vi "Log message.vi"(8 "error in (no error)":errorcluster, 9 "log level":u16(ring) items=[" STATUS ", " DEBBUG ", "  INFO  ", "WARNING ", " ERROR  ", "CRITICAL"], 10 "String":string, 11 "Channel in":refnum<class "Channel.lvclass">) -> (0 "error out":errorcluster, 3 "Channel out":refnum<class "Channel.lvclass">)   [LabVIEW 2018, in "Channel.lvclass"]
uses:
  Channel.lvclass
  Channel.lvclass/Channel.ctl
  Log File/Log File.lvclass
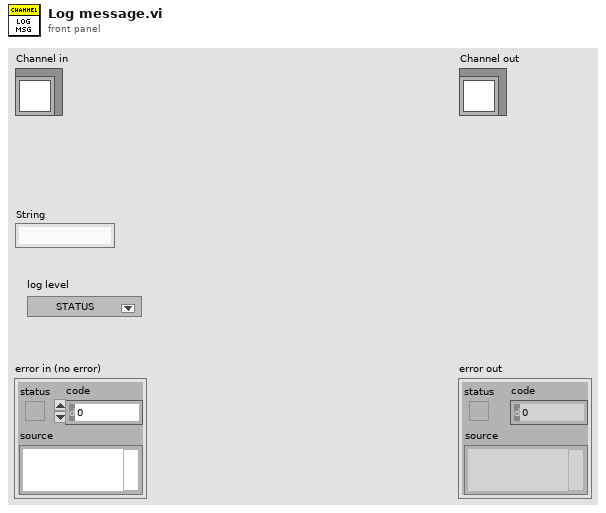
[diagram p1: front panel]
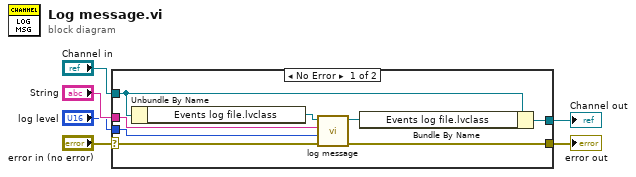
[diagram p0: block diagram]
diagram:
  n1 = case shown="No Error" "error in (no error)" {
    selector: "error in (no error)" -> [w10 w16]
    tunnel: [w9 w16] -> w5
    tunnel: [w11 w15] -> w3
    tunnel: "Channel in" -> [w12 w15]
    tunnel: "String" -> [w8 _]
    tunnel: "log level" -> [w7 _]
    frame No Error {
      n2 = Unbundle By Name(w12) -> ("Events log file.lvclass"=w14:refnum<class "Log File.lvclass">)
      n3 = call-dynamic "log message.vi"("error in (no error)"=w10, "log level"=w7, "Message to log"=w8, "Log File in"=w14) -> ("error out"=w9:errorcluster, "Log File out"=w13:refnum<class "Log File.lvclass">)  [unwired: 6 in]
      n4 = Bundle By Name(cluster=w12, "Events log file.lvclass"=w13) -> (w11:refnum<class "Channel.lvclass">)
    }
    frame Error {
    }
  }
  "error out" <- w5
  "Channel out" <- w3
